vi "Configure.vi"(8 "error in (no error)":errorcluster, 11 "StageSPIM in":refnum<class "StageSPIM.lvclass">) -> (0 "error out":errorcluster, 2 "cancelled?":bool, 3 "StageSPIM out":refnum<class "StageSPIM.lvclass">)   [LabVIEW 2012, in "StageSPIM.lvclass"]
doc: "The configure method configures the details for the RabbitMQ connection. \n\nIn the derived class, make a call to the parent for setting these parameters."
uses:
  StageSPIM.lvclass
  connection_type.ctl
  baud_rate_control.ctl
  port_control.ctl
  <vilib>/Utility/miscctls.llb/LVPointTypeDef.ctl
  StageSPIM.lvclass/StageSPIM.ctl
  <vilib>/Distrio/Murmex/Murmex/Murmex.lvclass
panel:
  in  "button::configure murmex":bool
  in  "button::ok":bool
  in  "button::cancel":bool
  in  "Tab Control":enum32{"Comport", "Stages", "Other"}(tab)
  in  "Port":T1 items=["COM1", "COM2", "COM3", "COM4", "COM5", "COM6", "COM7", "COM8", "COM9", "COM10", "COM11", "COM12", "COM13", "COM14", "COM15", "COM16", "COM17", "COM18", "COM19", "COM20", "COM21", "COM22", "COM23", "COM24", "COM25", "COM26", "COM27", "COM28", "COM29", "COM30"]
  in  "Baudrate":T2=3 items=["9600", "14400", "19200", "38400", "57600", "115200"]
  in  "Interface":T3=enum."USB_DaisyChain"
  in  "S/N Master controller":string
  in  "Update frequency":dbl[unit]
  in  "speedFocus":dbl[unit]
  in  "speedZ":dbl[unit]
  in  "speedY":dbl[unit]
  in  "speedX":dbl[unit]
  in  "speedA":dbl[unit]
  in  "soft min limit":dbl[](array[numeric])
  in  "soft max limit":dbl[](array[numeric])
  in  "Reporting folder":path
  in  "Autofocus component":string
  # "startup speed"
  # "A"
  # "X"
  # "Y"
  # "Z"
  # "Focus"
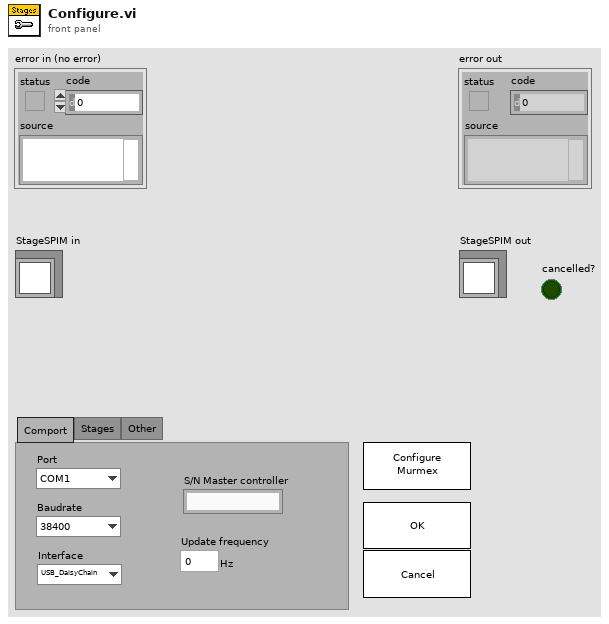
[diagram p1: front panel]
types:
  T1 = typedef "StageSPIM.lvclass/port_control.ctl" = i32
  T2 = typedef "StageSPIM.lvclass/baud_rate_control.ctl" = u16
  T3 = typedef "StageSPIM.lvclass/connection_type.ctl" = enum16{"RS232", "RS232 DaisyChain", "USB", "USB_DaisyChain"}
  T4 = typedef "LVPointTypeDef.ctl" = cluster{"Horizontal":i16, "Vertical":i16}
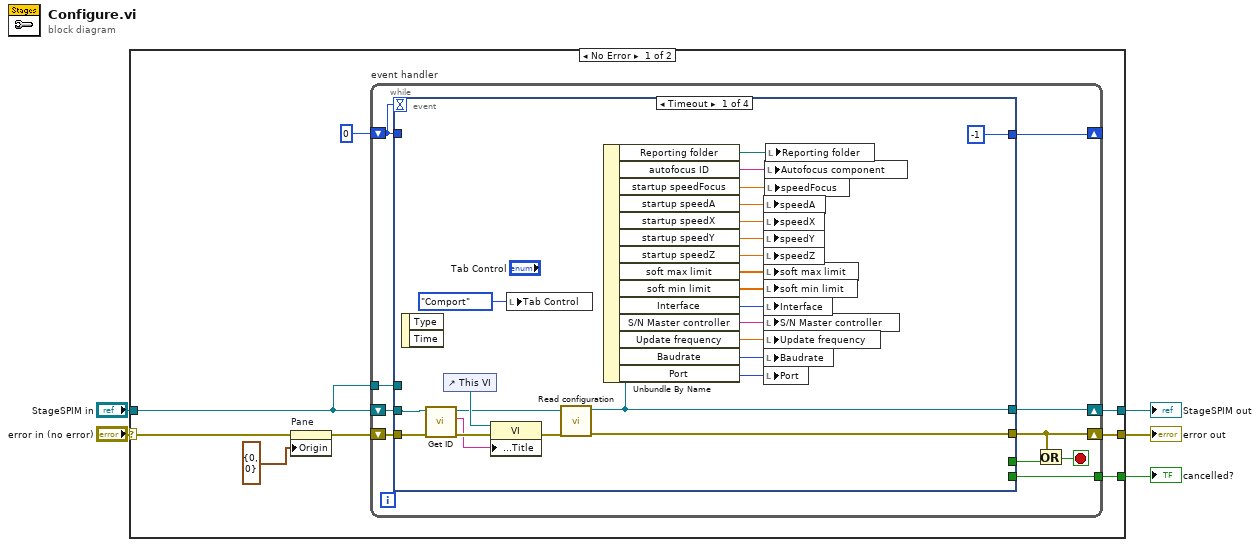
[diagram p0: block diagram]
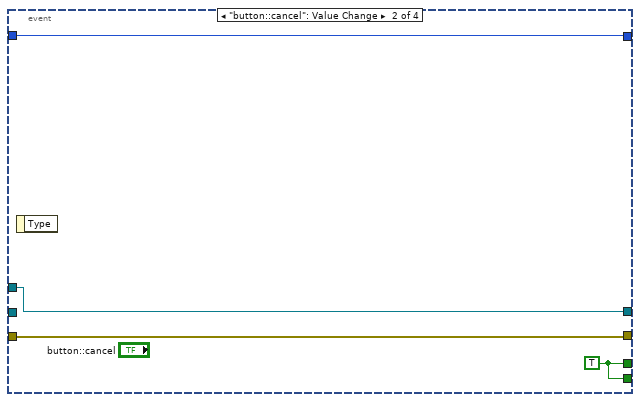
[diagram p2: hidden frame]
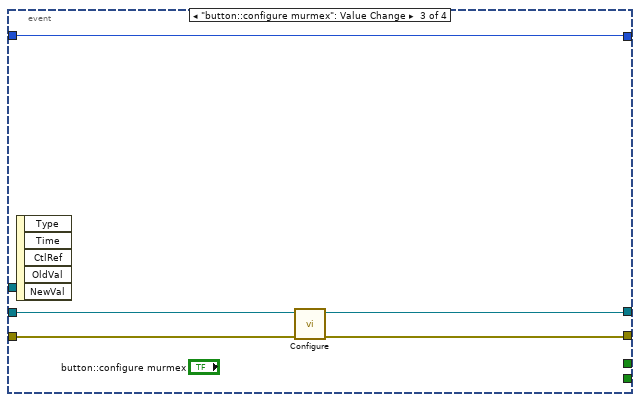
[diagram p3: hidden frame]
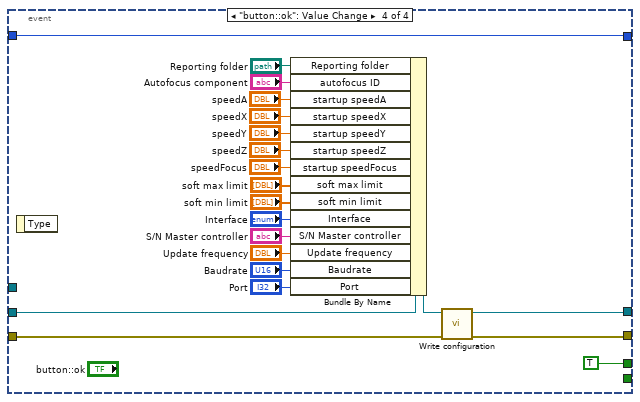
[diagram p4: hidden frame]
diagram:
  n1 = case shown="No Error" "error in (no error)" {
    selector: "error in (no error)" -> [w13 w79]
    tunnel: "StageSPIM in" -> [w10 w80]
    tunnel: [w8 w79] -> w3
    tunnel: [w7 w80] -> w2
    tunnel: [w6 _] -> w1
    frame No Error {
      n2 = property on="Pane" class="Pane"(error in=w13, "Origin"=T4 {"Horizontal"=0, "Vertical"=0}) -> (error out=w9:errorcluster)  [unwired: 1 in, 1 out]
      n3 = while "event handler" {
        shift-right: [w18] -> _
        shift-left: 0 -> [w23]
        shift-right: [w19] -> w7
        shift-left: w10 -> [w22]
        tunnel: w10 -> [w21]
        shift-right: [w16] -> w8
        shift-left: w9 -> [w20]
        tunnel: [w14] -> w6
        stop <- w17 stop-if-true
        n4 = event shown="[0] Timeout" {
          selector: _ -> [_ _ _ _]
          dyn-events: _ -> [_ _ _ _]
          timeout: w23 -> [_ _ _ _]
          tunnel: w23 -> [_ w49 w53 w72]
          tunnel: w22 -> [w44 _ w55 w76]
          tunnel: w21 -> [_ w50 _ _]
          tunnel: w20 -> [w48 w52 w57 w78]
          tunnel: [w40 w50 w54 w74] -> w19
          tunnel: [w41 w52 w56 w77] -> w16
          tunnel: [-1 w49 w53 w72] -> w18
          tunnel: [_ w51 _ TRUE ("force loading?")] -> w15
          tunnel: [_ w51 _ _] -> w14
          event Timeout {
            n5 = event-data() -> ()  [unwired: 1 in, 2 out]
            n6 = call <vilib>:"Get ID.vi"("error in (no error)"=w48, "Murmex in"=w44) -> ("error out"=w47:errorcluster, "component id"=w45:string, "Murmex out"=w42:refnum<class "StageSPIM.lvclass">)  [unwired: 7 in]
            n7 = control-ref of="This VI"() -> (w46:refnum<vi>)
            n8 = property class="VI"(reference=w46, error in=w47, "Front Panel.Title"=w45) -> (error out=w43:errorcluster)  [unwired: 1 out]
            n9 = local write "Tab Control"(enum32{"Comport", "Stages", "Other"}."Comport" ("Tab Control")) -> ()
            n10 = call <vilib>:"Read configuration.vi"("error in (no error)"=w43, "Murmex in"=w42) -> ("error out"=w41:errorcluster, "Murmex out"=w40:refnum<class "StageSPIM.lvclass">)  [unwired: 7 in, 1 out]
            n11 = Unbundle By Name(w40) -> ("Reporting folder"=w24:path, "autofocus ID"=w25:string, "startup speedFocus"=w27:dbl[unit], "startup speedA"=w31:dbl[unit], "startup speedX"=w30:dbl[unit], "startup speedY"=w29:dbl[unit], "startup speedZ"=w28:dbl[unit], "soft max limit"=w38:dbl[], "soft min limit"=w37:dbl[], "Interface"=w36:T3, "S/N Master controller"=w35:string, "Update frequency"=w34:dbl[unit], "Baudrate"=w33:T2, "Port"=w32:T1)
            n12 = local write "speedA"(w31) -> ()
            n13 = local write "speedX"(w30) -> ()
            n14 = local write "speedY"(w29) -> ()
            n15 = local write "speedZ"(w28) -> ()
            n16 = local write "soft max limit"(w38) -> ()
            n17 = local write "soft min limit"(w37) -> ()
            n18 = local write "Interface"(w36) -> ()
            n19 = local write "S/N Master controller"(w35) -> ()
            n20 = local write "Update frequency"(w34) -> ()
            n21 = local write "Baudrate"(w33) -> ()
            n22 = local write "Port"(w32) -> ()
            n23 = local write "Autofocus component"(w25) -> ()
            n24 = local write "speedFocus"(w27) -> ()
            n25 = local write "Reporting folder"(w24) -> ()
          }
          event "button::cancel": Value Change {
            w51 = TRUE ("force loading?")
            n26 = event-data() -> ()  [unwired: 1 in, 1 out]
          }
          event "button::configure murmex": Value Change {
            n27 = event-data() -> ()  [unwired: 1 in, 5 out]
            n28 = call-parent "Configure.vi"("error in (no error)"=w57, "Murmex in"=w55) -> ("error out"=w56:errorcluster, "Murmex out"=w54:refnum<class "StageSPIM.lvclass">)  [unwired: 7 in, 1 out]
          }
          event "button::ok": Value Change {
            n29 = event-data() -> ()  [unwired: 1 in, 1 out]
            n30 = Bundle By Name(cluster=w76, "Reporting folder"="Reporting folder", "autofocus ID"="Autofocus component", "startup speedA"="speedA", "startup speedX"="speedX", "startup speedY"="speedY", "startup speedZ"="speedZ", "startup speedFocus"="speedFocus", "soft max limit"="soft max limit", "soft min limit"="soft min limit", "Interface"="Interface", "S/N Master controller"="S/N Master controller", "Update frequency"="Update frequency", "Baudrate"="Baudrate", "Port"="Port") -> (w75:refnum<class "StageSPIM.lvclass">)
            n31 = call <vilib>:"Write configuration.vi"("error in (no error)"=w78, "Murmex in"=w75) -> ("error out"=w77:errorcluster, "Murmex out"=w74:refnum<class "StageSPIM.lvclass">)  [unwired: 8 in]
          }
        }
        n32 = Or(x=w16, y=w15) -> (x .or. y?=w17:bool)
      }
    }
    frame Error {
    }
  }
  "error out" <- w3
  "StageSPIM out" <- w2
  "cancelled?" <- w1
